vi "Keithley24xx_MeasVih.vi"(0 "VISA In":refnum<visa-resource-name>, 1 "Vol, V":dbl, 5 "VISA Out":refnum<visa-resource-name>, 7 "MeasF Out":string, 9 "Step, V":dbl, 11 "ErrIn In":errorcluster, 12 "Err Out":errorcluster, 13 "Begin Level, V":dbl, 14 "Vih, V":dbl) -> (4 "VISA Out 2":refnum<visa-resource-name>, 6 "VISA In 2":refnum<visa-resource-name>, 8 "Vih meas, В":dbl format="%#.3g", 10 "Err In":errorcluster, 15 "Err Out 2":errorcluster)   [LabVIEW 2014]
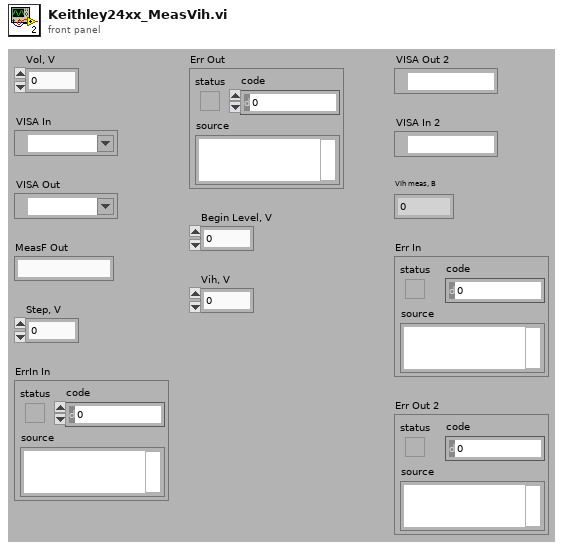
[diagram p1: front panel]
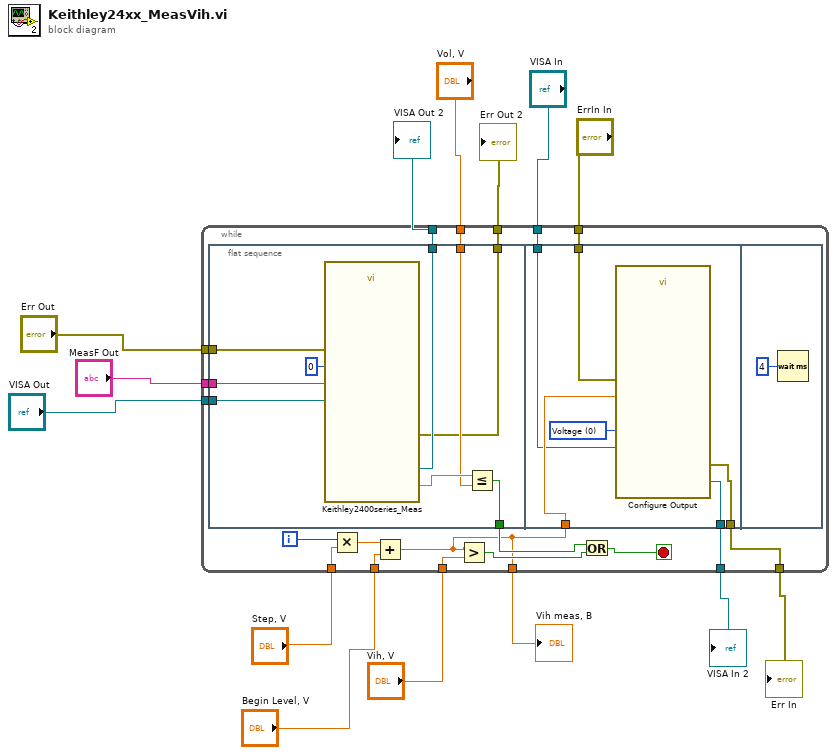
[diagram p0: block diagram]
diagram:
  n1 = while {
    tunnel: [w28] -> w7
    tunnel: "Err Out" -> [w27]
    tunnel: "MeasF Out" -> [w26]
    tunnel: "VISA Out" -> [w25]
    tunnel: "ErrIn In" -> [w24]
    tunnel: "VISA In" -> [w23]
    tunnel: "Step, V" -> [w22]
    tunnel: "Vih, V" -> [w21]
    tunnel: "Vol, V" -> [w20]
    tunnel: [w19] -> w9
    tunnel: [w18] -> w10
    tunnel: [w17] -> w11
    tunnel: [w16] -> w12
    tunnel: "Begin Level, V" -> [w15]
    i -> [w33]
    stop <- w29 stop-if-true
    n2 = flat-sequence {
      tunnel: [w41] -> w31
      tunnel: w27 -> [w39]
      tunnel: w26 -> [w38]
      tunnel: w25 -> [w37]
      tunnel: w20 -> [w36]
      tunnel: [w35] -> w19
      tunnel: [w34] -> w16
      tunnel: w28 -> [w47]
      tunnel: w24 -> [w46]
      tunnel: w23 -> [w45]
      tunnel: [w44] -> w18
      tunnel: [w43] -> w17
      frame #0 {
        n3 = call "Keithley2400series_Meas.vi"("MEAS:<f>"=w38, "error in (no error)"=w39, "MEAS mode, 0 Volt"=u16 0, "VISA resource name in"=w37) -> ("error out"=w34:errorcluster, "Замер"=w42:dbl, "VISA out"=w35:refnum<visa-resource-name>)  [unwired: 1 in, 1 out]
        n4 = Less Or Equal?(x=w42, y=w36) -> (x <= y?=w41:bool)
      }
      frame #1 {
        w48 = u16 0 items=["Voltage", "Current"] ("Source Mode  (0: Voltage)")
        n5 = call "Configure Output.vi"("Source Mode  (0: Voltage)"=w48, "error in (no error)"=w46, "Output Level (0)"=w47, "VISA resource name"=w45) -> ("error out"=w43:errorcluster, "VISA resource name out"=w44:refnum<visa-resource-name>)  [unwired: 6 in]
      }
      frame #2 {
        n6 = Wait (ms)(milliseconds to wait=u32 4) -> ()  [unwired: 1 out]
      }
    }
    n7 = Multiply(x=w33, y=w22) -> (x*y=w32:dbl)
    n8 = Add(x=w32, y=w15) -> (x+y=w28:dbl)
    n9 = Greater?(x=w28, y=w21) -> (0:w30:bool)
    n10 = Or(x=w31, y=w30) -> (x .or. y?=w29:bool)
  }
  "Vih meas, В" <- w7
  "VISA Out 2" <- w9
  "VISA In 2" <- w10
  "Err In" <- w11
  "Err Out 2" <- w12
